vi "_045.vi"() -> ()   [LabVIEW 2024]
panel:
  out "element":dbl
  in  "disabled index (row)":i32
  in  "disabled index (col) 2":i32
  out "subarray 2":dbl[](array[numeric])
  in  "disabled index (col)":i32
  in  "index (row)":i32
  out "subarray":dbl[](array[numeric])
  out "Waveform Graph 1":dbl[](graph)
  out "Graph 2":dbl[][](graph)
  out "size(s)":i32
  out "size(s) 2":i32[](array[numeric])
  in  "Array":dbl[](array[numeric])
  in  "Input 2":dbl
  out "A+B":bool[](array[boolean])
  out "A":bool[](array[boolean])
  in  "Input":dbl
  out "B":bool[](array[boolean])
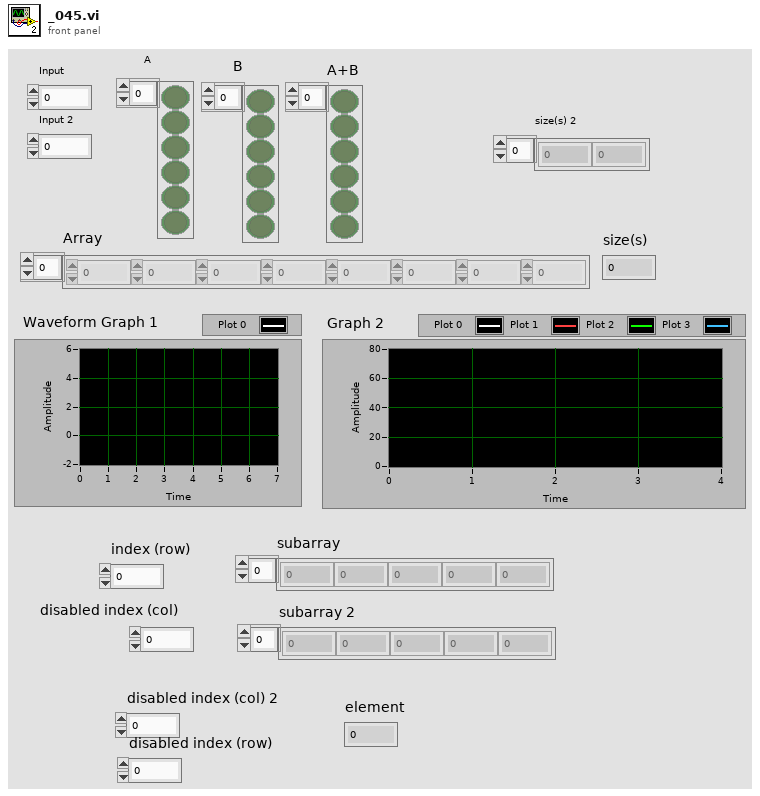
[diagram p1: front panel]
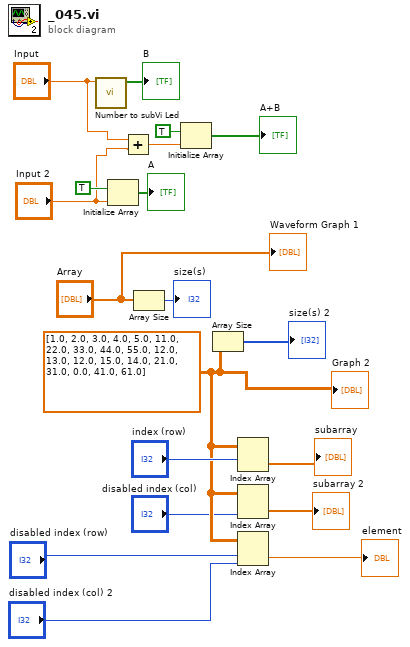
[diagram p0: block diagram]
diagram:
  w6 = dbl[][] [[1.0, 2.0, 3.0, 4.0, 5.0], [11.0, 22.0, 33.0, 44.0, 55.0], [12.0, 13.0, 12.0, 15.0, 14.0], [21.0, 31.0, 0.0, 41.0, 61.0]] ("Array 2")
  n1 = call "Number to subVi Led.vi"("Input in"="Input") -> ("B"=→"B":bool[])  [unwired: 10 in]
  n2 = Initialize Array(TRUE, "Input 2") -> (→"A":bool[])
  n3 = Add(x="Input", y="Input 2") -> (x+y=w15:dbl)
  n4 = Array Size(array="Array") -> (size(s)=→"size(s)":i32)
  n5 = Initialize Array "Initialize Array"(TRUE, w15) -> (→"A+B":bool[])
  n6 = Array Size(array=w6) -> (size(s)=→"size(s) 2":i32[])
  n7 = Index Array "Index Array"(array=w6, index (row)="index (row)") -> (element=→"subarray":dbl[])  [unwired: 1 in]
  n8 = Index Array(array=w6, index (col)="disabled index (col)") -> (element=→"subarray 2":dbl[])  [unwired: 1 in]
  n9 = Index Array(array=w6, index (row)="disabled index (row)", index (col)="disabled index (col) 2") -> (element=→"element":dbl)
  "Graph 2" <- w6
  "Waveform Graph 1" <- "Array"
